vi "BiServer-10.vi"() -> ()   [LabVIEW 2024]
uses:
  <vilib>/Analysis/NI_AALBase.lvlib
panel:
  in  "?":bool
  in  "Port":u16
  in  ".NET Container":refnum<k24>(container)
  # "Instructions:\n1. Open the Simple Data Client.vi.\n2. Run this VI first.\n3. Run the Simple Data Client.vi\nsecond.\n4. Adjust the Function and # of Points\ncontrols to see the plot on the front\npanel of the Simple Data Client.vi\nchange."
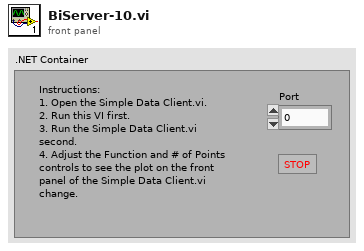
[diagram p1: front panel]
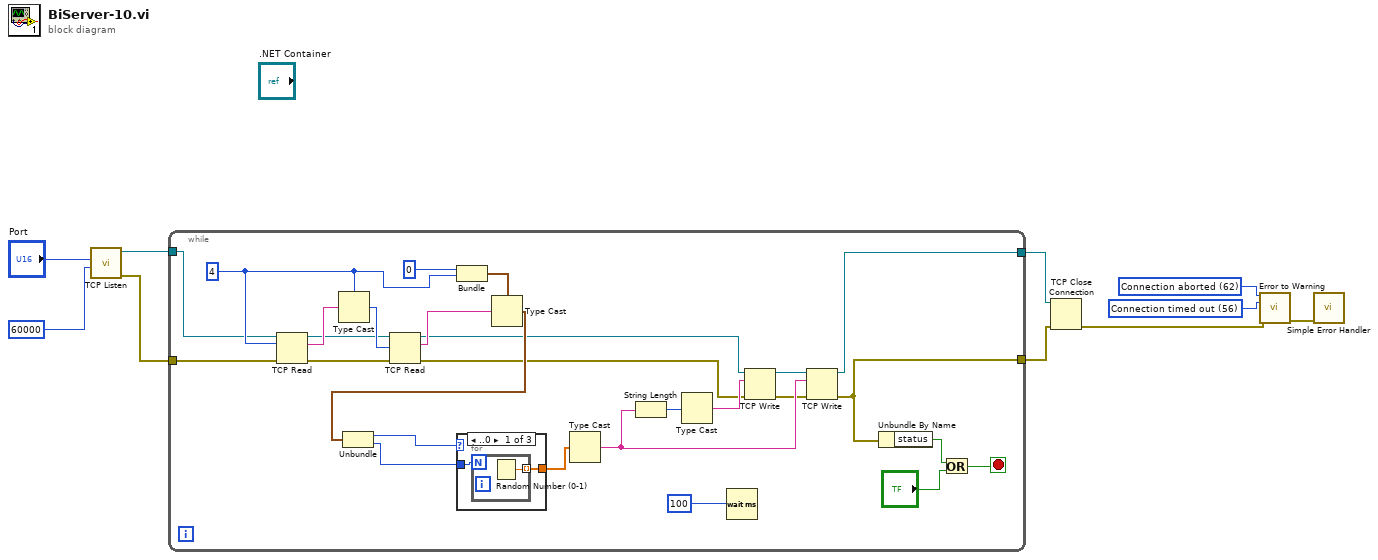
[diagram p0: block diagram]
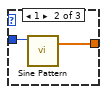
[diagram p2: hidden frame]
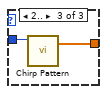
[diagram p3: hidden frame]
diagram:
  w2 = 56 items=["No Error", "Argument Error", "Memory Full", "Out of Zone", "End of File", "File Already Open", "Generic File IO Error", "File Not Found", "File Permission Error", "Disk Full", "Duplicate Path", "Too Many Files Open", "Not Enabled", "Resource File Not Found", "Cannot Add Resource", "Resource Not Found", "Image Not Found", "Image Memory Error", "Pen Does Not Exist", "Config Bad Type", "Config Token Not Found", "Config Parse Error", "Config Memory Error", "Bad External Code Format", "Bad External Code Offset", "External Code Not Present", "Null Window", "Destroy Window Mixup", "Null Menu", "Print Aborted", "Bad Print Record", "Print Driver Error", "Windows Error During Print", "Memory Error During Print", "Print Dialog Error", "Generic Print Error", "Invalid Device Refnum", "Device Not Found", "Device Parameter Error", "Device Unit Error", "Can't Open Device", "Device Call Aborted", "Generic Error", "Cancelled By User", "Object ID Too Low", "Object ID Too High", "Object Not In Heap", "Unknown Heap", "Bad DefProc ID", "DefProc Not In Table", "Message Out Of Range", "Null Method", "Unknown Message", "Manager Call Not Supported", "Bad address", "Connection In progress", "Connection timed out", "Connection is already in progress", "Network attribute not supported", "Network error", "Address in use", "System out of memory", "Connection aborted", "Connection refused", "Connection is not connected", "Connection is already connected", "Connection closed", "Initialize error (interapplication manager)", "Bad occurrence", "Wait on unbound occurrence handler", "Occurrence queue overflow", "Bad path", "Semaphore not signaled", "Unrecognized type (interapplication manager)"] ("2nd Error to Convert")
  w3 = 62 items=["No Error", "Argument Error", "Memory Full", "Out of Zone", "End of File", "File Already Open", "Generic File IO Error", "File Not Found", "File Permission Error", "Disk Full", "Duplicate Path", "Too Many Files Open", "Not Enabled", "Resource File Not Found", "Cannot Add Resource", "Resource Not Found", "Image Not Found", "Image Memory Error", "Pen Does Not Exist", "Config Bad Type", "Config Token Not Found", "Config Parse Error", "Config Memory Error", "Bad External Code Format", "Bad External Code Offset", "External Code Not Present", "Null Window", "Destroy Window Mixup", "Null Menu", "Print Aborted", "Bad Print Record", "Print Driver Error", "Windows Error During Print", "Memory Error During Print", "Print Dialog Error", "Generic Print Error", "Invalid Device Refnum", "Device Not Found", "Device Parameter Error", "Device Unit Error", "Can't Open Device", "Device Call Aborted", "Generic Error", "Cancelled By User", "Object ID Too Low", "Object ID Too High", "Object Not In Heap", "Unknown Heap", "Bad DefProc ID", "DefProc Not In Table", "Message Out Of Range", "Null Method", "Unknown Message", "Manager Call Not Supported", "Bad address", "Connection In progress", "Connection timed out", "Connection is already in progress", "Network attribute not supported", "Network error", "Address in use", "System out of memory", "Connection aborted", "Connection refused", "Connection is not connected", "Connection is already connected", "Connection closed", "Initialize error (interapplication manager)", "Bad occurrence", "Wait on unbound occurrence handler", "Occurrence queue overflow", "Bad path", "Semaphore not signaled", "Unrecognized type (interapplication manager)"] ("1st Error to Convert")
  n1 = call <vilib>:"TCP Listen.vi"("timeout ms (wait forever: -1)"=60000, "port"="Port") -> ("error out"=w8:errorcluster, "connection ID"=w7:refnum<k5>)  [unwired: 5 in, 3 out]
  n2 = while {
    tunnel: w8 -> [w21]
    tunnel: w7 -> [w23]
    tunnel: [w14] -> w6
    tunnel: [w17] -> w5
    stop <- w26 stop-if-true
    w35 = 4
    n3 = TCP Read(connection ID=w23, bytes to read=w35, error in (no error)=w21) -> (connection ID out=w22:refnum<k5>, data out=w34:string, error out=w20:errorcluster)  [unwired: 2 in]
    n4 = Type Cast(type=w35, x=w34) -> (*(type *) &x=w33:i32)
    n5 = TCP Read(connection ID=w22, bytes to read=w33, error in (no error)=w20) -> (connection ID out=w16:refnum<k5>, data out=w31:string, error out=w19:errorcluster)  [unwired: 2 in]
    n6 = Bundle(u16 0, w35) -> (w32:cluster{u16, i32})  [unwired: 1 in]
    n7 = Type Cast(type=w32, x=w31) -> (*(type *) &x=w30:cluster{u16, i32})
    n8 = Unbundle(w30) -> (w12:u16, w11:i32)
    n9 = case shown="..0" w12 {
      tunnel: w11 -> [w39 w42 w44]
      tunnel: [w38 w41 w43] -> w13
      frame ..0 {
        n10 = for {
          N: w39 -> [_]
          tunnel: [w40] -> w38 mode=indexing
          n11 = Random Number (0-1)() -> (number: 0 to 1=w40:dbl)
        }
      }
      frame 1 {
        n12 = call <vilib>:"Sine Pattern.vi"("samples"=w42) -> ("Sinusoidal Pattern"=w41:dbl[])  [unwired: 3 in, 1 out]
      }
      frame 2.. {
        n13 = call <vilib>:"Chirp Pattern.vi"("samples"=w44) -> ("Chirp Pattern"=w43:dbl[])  [unwired: 3 in, 1 out]
      }
    }
    n14 = Type Cast(x=w13) -> (*(type *) &x=w27:string)  [unwired: 1 in]
    n15 = String Length(string=w27) -> (length=w28:i32)
    n16 = Type Cast(x=w28) -> (*(type *) &x=w29:string)  [unwired: 1 in]
    n17 = Wait (ms)(milliseconds to wait=100) -> ()  [unwired: 1 out]
    n18 = TCP Write(connection ID=w16, data in=w29, error in (no error)=w19) -> (connection ID out=w15:refnum<k5>, error out=w18:errorcluster)  [unwired: 1 in, 1 out]
    n19 = TCP Write(connection ID=w15, data in=w27, error in (no error)=w18) -> (connection ID out=w14:refnum<k5>, error out=w17:errorcluster)  [unwired: 1 in, 1 out]
    n20 = Unbundle By Name(w17) -> ("status"=w24:bool)
    n21 = Or(x=w24, y="?") -> (x .or. y?=w26:bool)
  }
  n22 = TCP Close Connection(connection ID=w6, error in (no error)=w5) -> (error out=w4:errorcluster)  [unwired: 1 in, 1 out]
  n23 = call <vilib>:"Error to Warning.vi"("1st Error to Convert"=w3, "2nd Error to Convert"=w2, "error in"=w4) -> ("warning out"=w1:errorcluster)  [unwired: 12 in]
  n24 = call <vilib>:"Simple Error Handler.vi"("error in (no error)"=w1) -> ()  [unwired: 4 in, 5 out]
